vi "set_amplif_boe.vi"(8 "error in (no error)":errorcluster, 10 "ParamIn":i32, 11 "app_data in":T1) -> (0 "error out":errorcluster, 3 "app_data out":T1)   [LabVIEW 2017]
uses:
  controls/app_data.ctl
  controls/instruments.ctl
  Unicorn Labview Library/Control/unicorn_Param.ctl
  Unicorn Labview Library/Control/unicorn_conn.ctl
  Unicorn Labview Library/Control/unicorn_JSON.ctl
  Unicorn Labview Library/Control/unicorn_ParamInt.ctl
  Unicorn Labview Library/Control/unicorn_Telemetry.ctl
  Unicorn Labview Library/Control/unicorn_Table.ctl
  Unicorn Labview Library/Control/unicorn_ParamFloat.ctl
  Unicorn Labview Library/Unicorn Library.lvlib
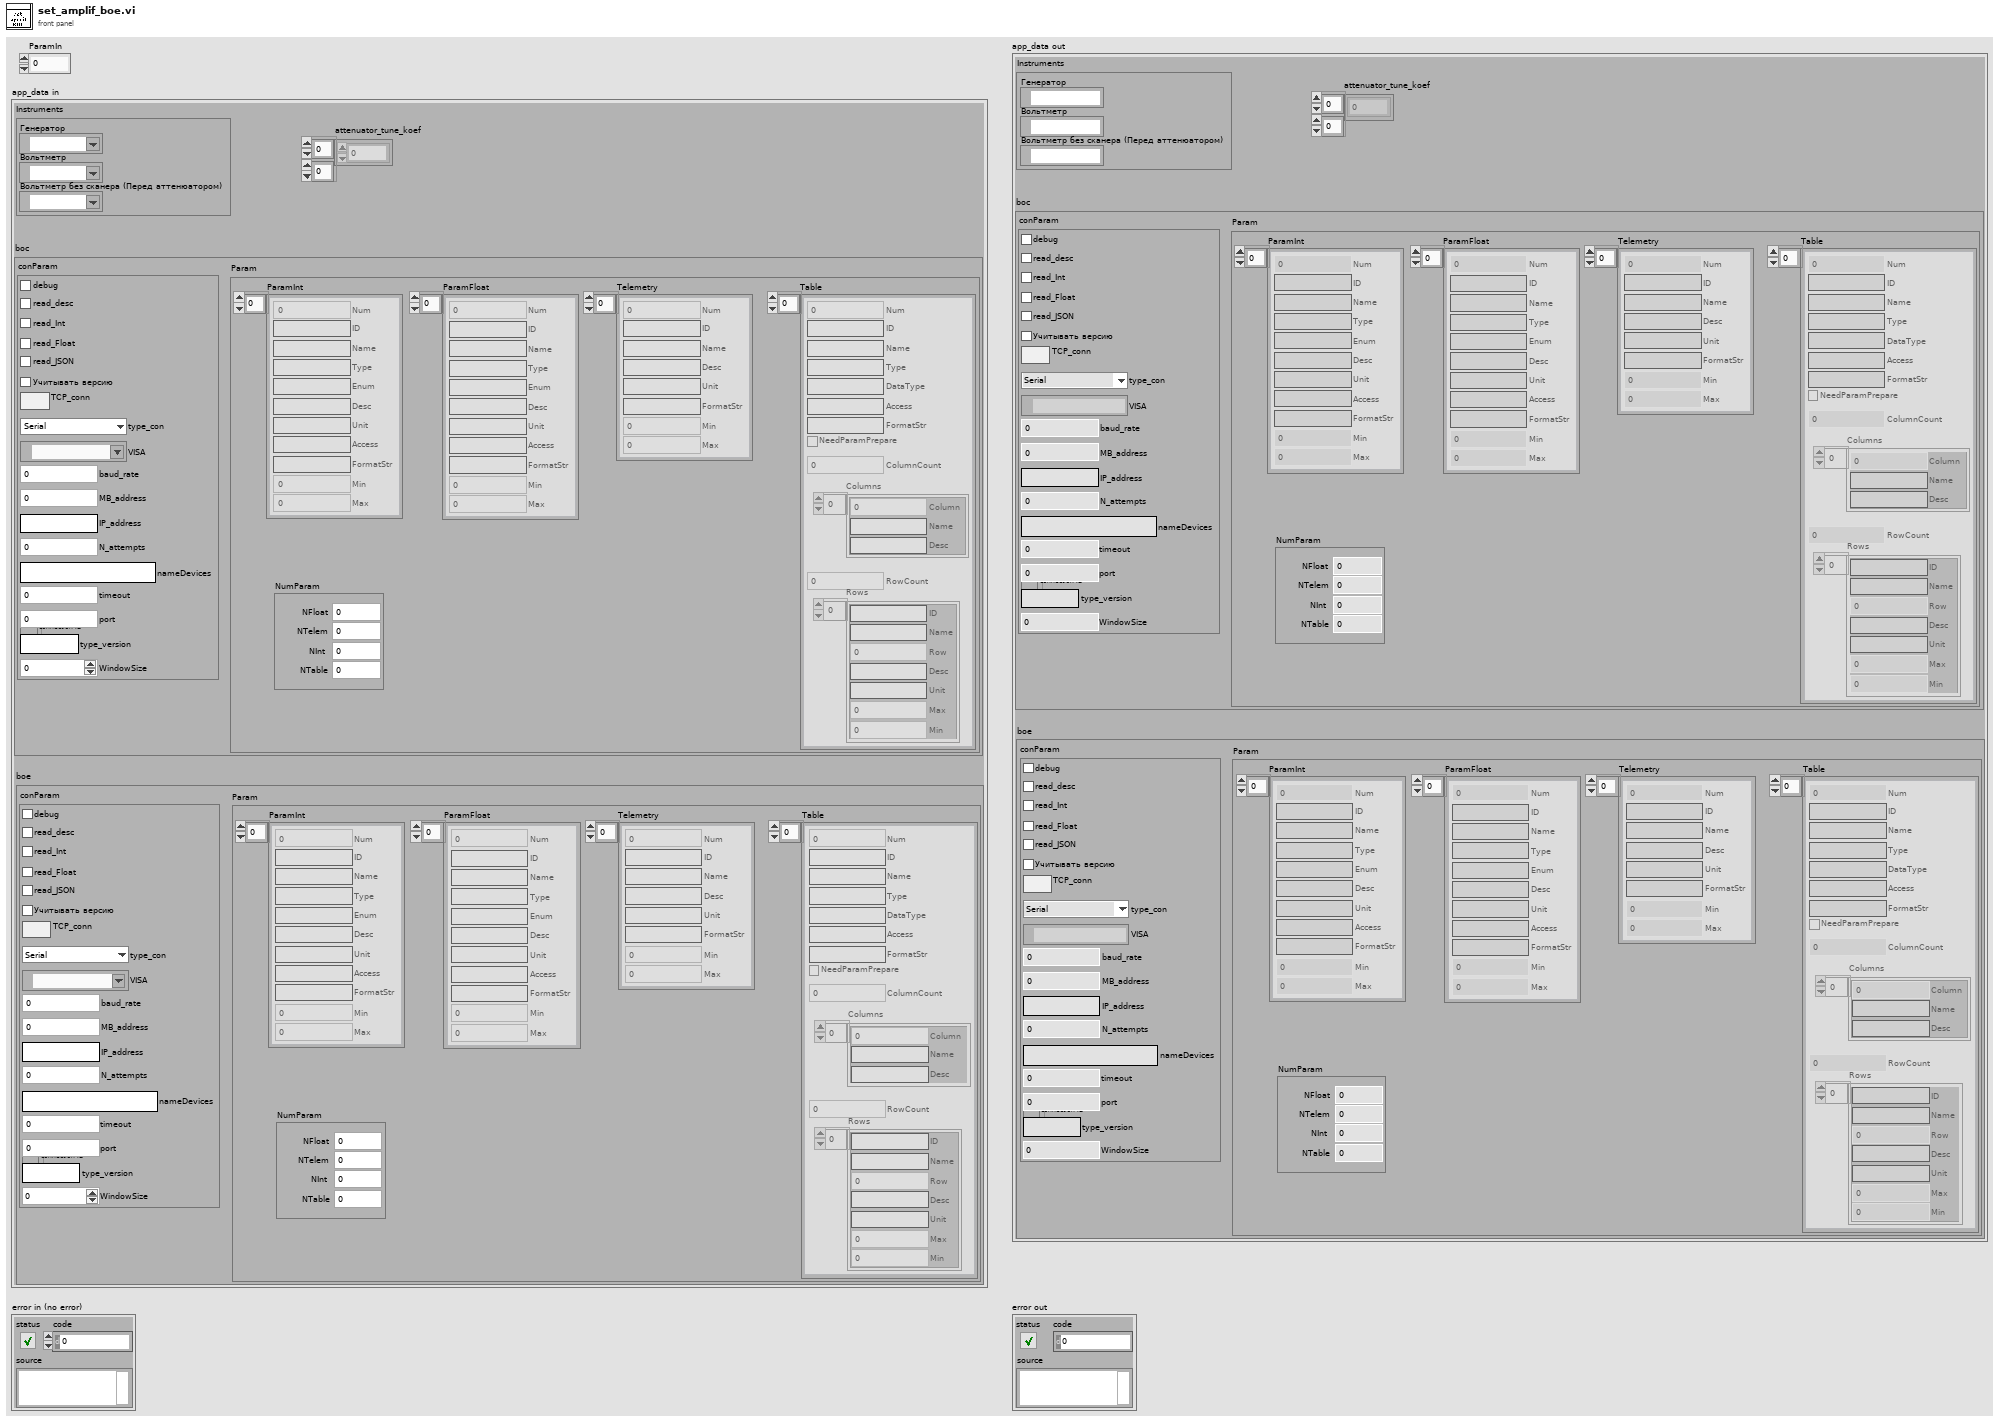
[diagram p1: front panel]
types:
  T1 = typedef "app_data.ctl" = cluster{"Instruments":T2, "boc":T3, "boe":T3, "attenuator_tune_koef":dbl[][]}
  T2 = typedef "instruments.ctl" = cluster{"generator":refnum<visa-resource-name>, "voltment_with_scaner":refnum<visa-resource-name>, "voltment_without_scaner":refnum<visa-resource-name>}
  T3 = typedef "Unicorn Library.lvlib/unicorn_Param.ctl" = cluster{"conParam":T4, "Param":T5}
  T4 = typedef "Unicorn Library.lvlib/unicorn_conn.ctl" = cluster{"ReadIntParam":bool, "ReadDescrParam":bool, "ReadFloatParam":bool, "debug":bool, "ReadJSON":bool, "IP_address":string, "N_attempts":i32, "type_con":enum16{"Serial", "TCP"}, "MB_address":i32, "VISA":refnum<visa-resource-name>, "connection ID":refnum<k5>, "nameDevices":string, "timeout":i32, "port":u16, "type_version":string, "baud_rate":u32, "VersionControl":bool, "TCP_conn":bool, "WindowSize":i32}
  T5 = typedef "Unicorn Library.lvlib/unicorn_JSON.ctl" = cluster{"NumParam":cluster{"NTelem":i32, "NInt":i32, "NFloat":i32, "NTable":i32}, "ParamInt":T6, "Telemetry":T7, "Table":T8, "ParamFloat":T9}
  T6 = typedef "Unicorn Library.lvlib/unicorn_ParamInt.ctl" = cluster{"ID":string, "Num":i32, "Name":string, "Type":string, "Enum":string, "Desc":string, "Unit":string, "Access":string, "FormatStr":string, "Min":i32, "Max":i32}[]
  T7 = typedef "Unicorn Library.lvlib/unicorn_Telemetry.ctl" = cluster{"ID":string, "Num":i32, "Name":string, "Desc":string, "Unit":string, "FormatStr":string, "Min":i32, "Max":i32}[]
  T8 = typedef "Unicorn Library.lvlib/unicorn_Table.ctl" = cluster{"Num":i32, "Access":string, "ColumnCount":i32, "NeedParamPrepare":bool, "Columns":cluster{"Column":i32, "Desc":string, "Name":string}[], "DataType":string, "FormatStr":string, "ID":string, "Name":string, "RowCount":i32, "Rows":cluster{"Desc":string, "ID":string, "Max":i32, "Min":i32, "Name":string, "Row":i32, "Unit":string}[], "Type":string}[]
  T9 = typedef "Unicorn Library.lvlib/unicorn_ParamFloat.ctl" = cluster{"ID":string, "Num":i32, "Name":string, "Type":string, "Enum":string, "Desc":string, "Unit":string, "Access":string, "FormatStr":string, "Min":i32, "Max":i32}[]
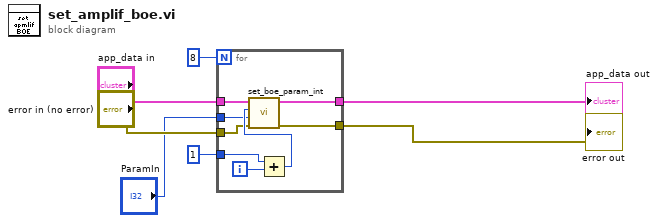
[diagram p0: block diagram]
diagram:
  n1 = for {
    N: 8 -> [_]
    tunnel: 1 -> [w14]
    tunnel: "app_data in" -> [w12]
    tunnel: "error in (no error)" -> [w11]
    tunnel: [w10] -> w6
    tunnel: [w9] -> w7
    tunnel: "ParamIn" -> [w8]
    i -> [w15]
    n2 = Add(x=w14, y=w15) -> (x+y=w13:i32)
    n3 = call "set_boe_param_int.vi"("error in (no error)"=w11, "ParamIn"=w8, "NumParamIn"=w13, "app_data in"=w12) -> ("error out"=w9:errorcluster, "app_data out"=w10:T1)  [unwired: 6 in]
  }
  "error out" <- w7
  "app_data out" <- w6
